vi "Create host uri prefix.vi"(8 "error in (no error)":errorcluster, 11 "address":string) -> (0 "error out":errorcluster, 3 "host uri prefix":string)   [LabVIEW 2015, in "RT Management.lvlib" / "WebDAV.lvclass"]
uses:
  WebDAV.lvclass
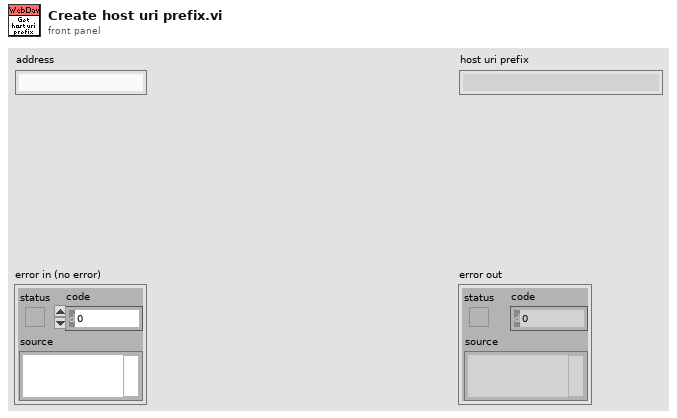
[diagram p1: front panel]
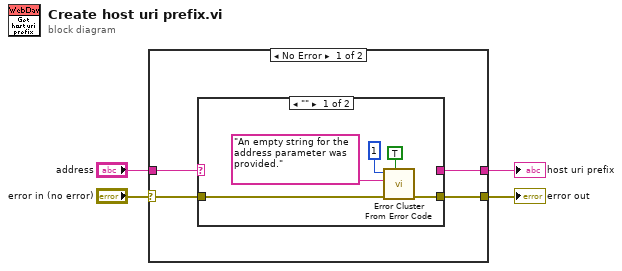
[diagram p0: block diagram]
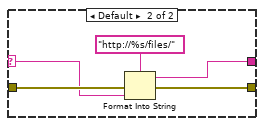
[diagram p2: hidden frame]
diagram:
  n1 = case shown="No Error" "error in (no error)" {
    selector: "error in (no error)" -> [w8 w19]
    tunnel: [w7 w19] -> w3
    tunnel: "address" -> [w5 _]
    tunnel: [w6 _] -> w1
    frame No Error {
      n2 = case shown="\"\"" w5 {
        selector: w5 -> [_ w14]
        tunnel: w8 -> [w13 w17]
        tunnel: [w12 w16] -> w7
        tunnel: [_ w15] -> w6
        frame "" {
          n3 = call <vilib>:"Error Cluster From Error Code.vi"("show call chain? (False)"=TRUE, "error in (no error)"=w13, "error message (\"\")"="An empty string for the address parameter was provided." ("error message (\"\")"), "error code (0)"=1) -> ("error out"=w12:errorcluster)  [unwired: 5 in]
        }
        frame Default {
          n4 = Format Into String(format string="http://%s/files/", error in=w17, w14) -> (resulting string=w15:string, error out=w16:errorcluster)  [unwired: 1 in]
        }
      }
    }
    frame Error {
    }
  }
  "error out" <- w3
  "host uri prefix" <- w1
